vi "Error Cluster.vi"() -> ()   [LabVIEW 2020]
uses:
  <vilib>/DAQmx/configure/timing.llb/DAQmx Timing (Sample Clock).vi
  <vilib>/DAQmx/read.llb/DAQmx Read (Analog DBL 1Chan 1Samp).vi
  <vilib>/DAQmx/create/channels.llb/DAQmx Create Channel (AI-Voltage-Basic).vi
panel:
  in  "error in 2":errorcluster
  out "error out 2":errorcluster
  out "error out 1":errorcluster
  in  "error in 1":errorcluster
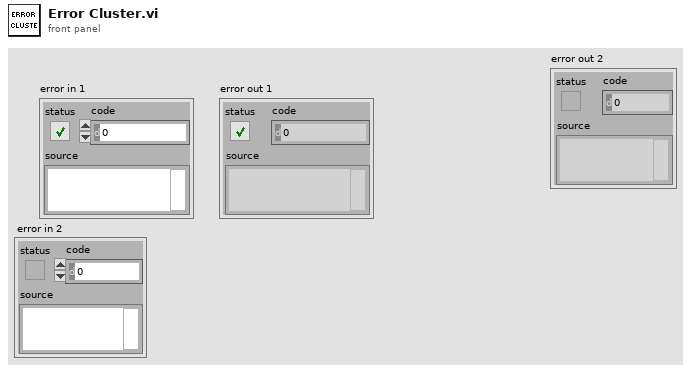
[diagram p1: front panel]
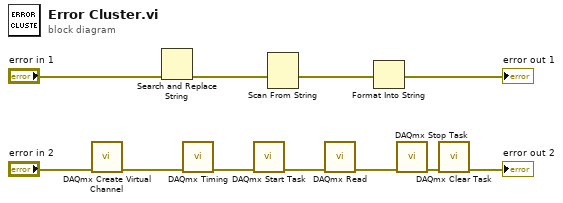
[diagram p0: block diagram]
diagram:
  n1 = call-poly <vilib>:"DAQmx Create Virtual Channel.vi"("error in"="error in 2") -> ("error out"=w4:errorcluster)  [unwired: 13 in, 1 out]
  n2 = Search and Replace String(error in="error in 1") -> (error out=w10:errorcluster)  [unwired: 7 in, 3 out]
  n3 = call-poly <vilib>:"DAQmx Timing.vi"("error in"=w4) -> ("error out"=w3:errorcluster)  [unwired: 13 in, 1 out]
  n4 = call <vilib>:"DAQmx Start Task.vi"("error in"=w3) -> ("error out"=w7:errorcluster)  [unwired: 13 in, 1 out]
  n5 = Scan From String(error in=w10) -> (error out=w11:errorcluster)  [unwired: 5 in, 2 out]
  n6 = call-poly <vilib>:"DAQmx Read.vi"("error in"=w7) -> ("error out"=w6:errorcluster)  [unwired: 12 in, 2 out]
  n7 = Format Into String(error in=w11) -> (error out=→"error out 1":errorcluster)  [unwired: 3 in, 1 out]
  n8 = call <vilib>:"DAQmx Stop Task.vi"("error in"=w6) -> ("error out"=w5:errorcluster)  [unwired: 13 in, 1 out]
  n9 = call <vilib>:"DAQmx Clear Task.vi"("error in"=w5) -> ("error out"=→"error out 2":errorcluster)  [unwired: 14 in]
